vi "Write Right Child Node.vi"(8 "error in (no error)":errorcluster, 10 "Math Formula String Phrasing.lvclass":refnum<class "Math Formula String Phrasing.lvclass">, 11 "Formula Phrasing Binary Tree Node in":refnum<class "Formula Phrasing Binary Tree Node.lvclass">) -> (0 "error out":errorcluster, 3 "Formula Phrasing Binary Tree Node out":refnum<class "Formula Phrasing Binary Tree Node.lvclass">)   [LabVIEW 2024, in "Formula Phrasing Binary Tree Node.lvclass"]
uses:
  Formula Phrasing Binary Tree Node.lvclass
  Math Formula String Phrasing/Math Formula String Phrasing.lvclass
  Formula Phrasing Binary Tree Node.lvclass/Formula Phrasing Binary Tree Node.ctl
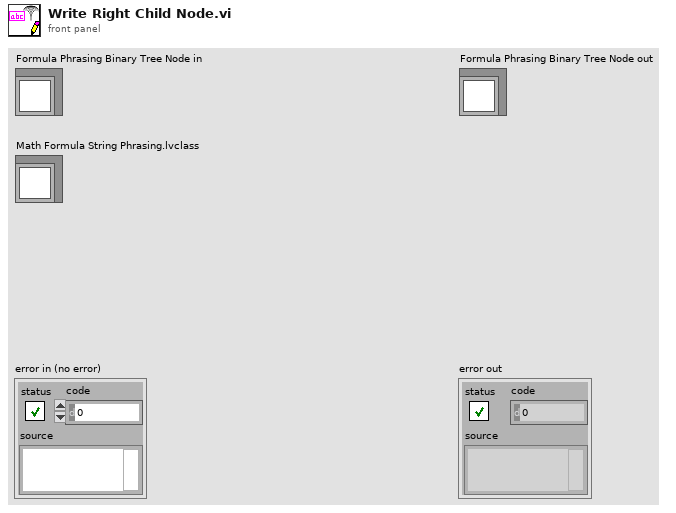
[diagram p1: front panel]
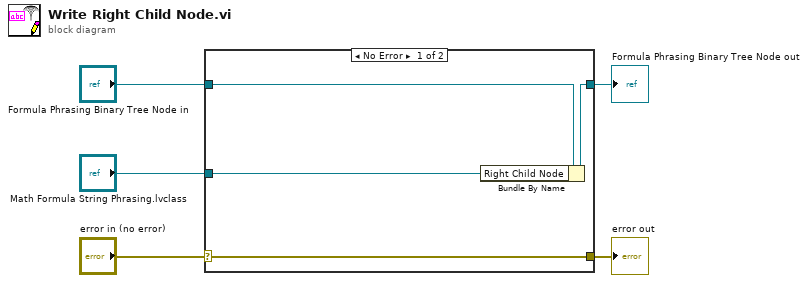
[diagram p0: block diagram]
diagram:
  n1 = case shown="No Error" "error in (no error)" {
    selector: "error in (no error)" -> [w9 w10]
    tunnel: [w9 w10] -> w4
    tunnel: [w7 w11] -> w2
    tunnel: "Formula Phrasing Binary Tree Node in" -> [w8 w11]
    tunnel: "Math Formula String Phrasing.lvclass" -> [w6 _]
    frame No Error {
      n2 = Bundle By Name(cluster=w8, "Right Child Node"=w6) -> (w7:refnum<class "Formula Phrasing Binary Tree Node.lvclass">)
    }
    frame Error {
    }
  }
  "error out" <- w4
  "Formula Phrasing Binary Tree Node out" <- w2
